vi "Remove Process.vi"(8 "error in (no error)":errorcluster, 10 "Process Name":string, 11 "Application In":refnum<class "Application.lvclass">) -> (0 "error out":errorcluster, 2 "App Process":refnum<class "Process.lvclass">, 3 "Application Out":refnum<class "Application.lvclass">)   [LabVIEW 2020, in "Application.lvclass"]
doc: "Get a specific process by name. A good pattern for using this VI is to wrap it with a string constant fed into the Process Name input and cast the received process to the expected process class. This pattern makes changing the class or the name easy as there is only one this single location where it is specified.\nThe VI can return processes from nested applications using the qualified name of the process."
uses:
  Application.lvclass
  C:/git/astemes-triarc-framework/source/Framework/Process/Process.lvclass
  Process/Process.lvclass
  C:/git/astemes-triarc-framework/source/Framework/Logging/Logging.lvclass
  Process/Process.lvclass/Process.ctl
  Application.lvclass/Application.ctl
  Process/Protected/Messaging/Request Message.vi
  <vilib>/AdvancedString/Delimited String to 1D String Array.vi
  Process/Protected/Messaging/Async Request Message.vi
  Process/Private/SubVIs/Handle Debug Data.vi
  Logging/Log Debug.vi
  <vilib>/AdvancedString/1D String Array to Delimited String.vi
  <vilib>/Utility/High Resolution Relative Seconds.vi
  Synchronous Request Callback/Synchronous Request Callback.lvclass
  C:/git/astemes-triarc-framework/source/Framework/Callback/Callback.lvclass
  <vilib>/Utility/error.llb/Error Cluster From Error Code.vi
  Synchronous Request Callback/Create.vi
  Process/Private/SubVIs/Wait for Response Message.vi
  Callback/Callback.lvclass
  Logging/Logging.lvclass
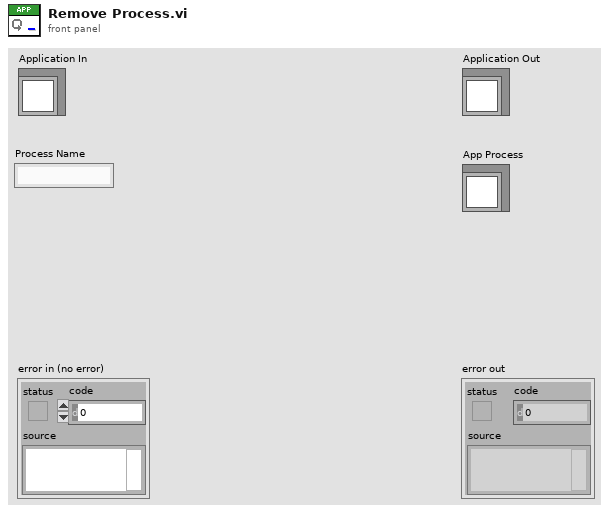
[diagram p1: front panel]
types:
  T1 = typedef "Process.lvclass/API Mode.ctl" = enum16{"Send Message", "Handle Message"}
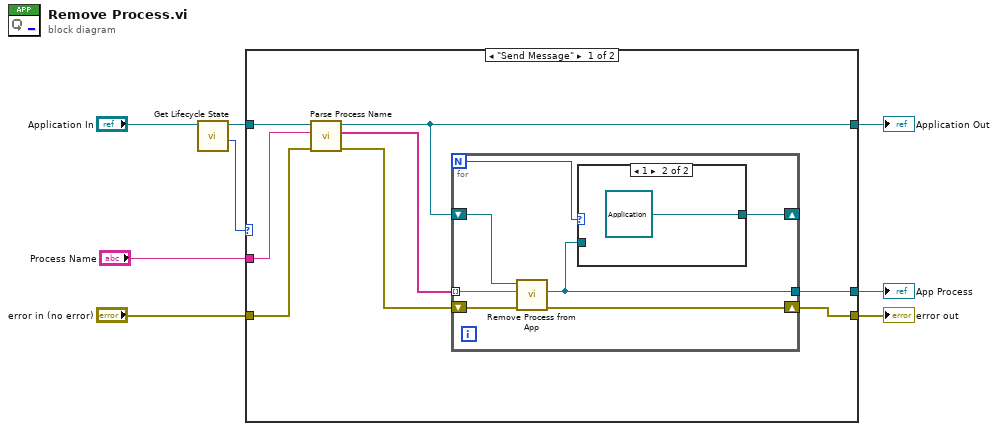
[diagram p0: block diagram]
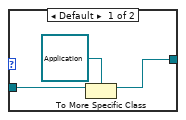
[diagram p2: hidden frame]
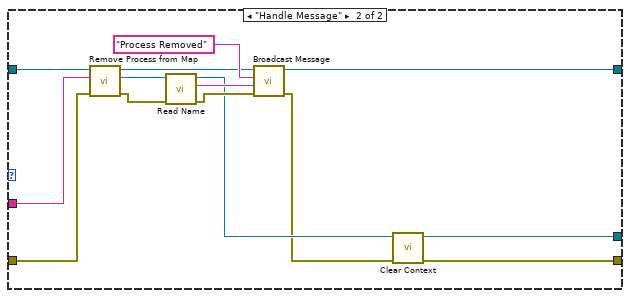
[diagram p3: hidden frame]
diagram:
  n1 = call "Get Lifecycle State.vi"("Process In"="Application In") -> ("API Mode"=w1:T1, "Process Out"=w2:refnum<class "Application.lvclass">)  [unwired: 7 in, 2 out]
  n2 = case shown="\"Send Message\"" w1 {
    tunnel: [w9 w31] -> w8
    tunnel: [w16 w28] -> w7
    tunnel: "Process Name" -> [w15 w41]
    tunnel: "error in (no error)" -> [w13 w32]
    tunnel: [w11 w35] -> w3
    tunnel: w2 -> [w10 w40]
    frame "Send Message" {
      n3 = call "Parse Process Name.vi"("error in (no error)"=w13, "Process Name"=w15, "Application In"=w10) -> ("error out"=w12:errorcluster, "Array"=w14:string[], "Application Out"=w11:refnum<class "Application.lvclass">)  [unwired: 6 in]
      n4 = for {
        N -> [w17]
        tunnel: [w19] -> w9
        tunnel: w14 -> [w21] mode=indexing
        shift-right: [w18] -> _
        shift-left: w11 -> [w22]
        shift-right: [w23] -> w16
        shift-left: w12 -> [w20]
        n5 = call "Remove Process from App.vi"("error in (no error)"=w20, "String"=w21, "Application In"=w22) -> ("error out"=w23:errorcluster, "Process"=w19:refnum<class "Process.lvclass">)  [unwired: 6 in, 1 out]
        n6 = case shown="1" w17 {
          tunnel: w19 -> [w26 _]
          tunnel: [w25 refnum<class "Application.lvclass"> refnum ("Application out")] -> w18
          frame Default {
            n7 = To More Specific Class(target class=refnum<class "Application.lvclass"> refnum ("Application out"), reference=w26) -> (specific class reference=w25:refnum<class "Application.lvclass">)  [unwired: 1 in, 1 out]
          }
          frame 1 {
          }
        }
      }
    }
    frame "Handle Message" {
      n8 = call "Remove Process from Map.vi"("error in (no error)"=w32, "Process Name"=w41, "Application In"=w40) -> ("error out"=w34:errorcluster, "Process"=w33:refnum<class "Process.lvclass">, "Application Out"=w36:refnum<class "Application.lvclass">)  [unwired: 6 in]
      n9 = call "Read Name.vi"("error in (no error)"=w34, "Process In"=w33) -> ("error out"=w38:errorcluster, "Qualified Name"=w37:string, "Process Out"=w30:refnum<class "Process.lvclass">)  [unwired: 6 in, 1 out]
      n10 = call-dynamic "Broadcast Message.vi"("error in (no error)"=w38, "Message Data"=w37, "Message"="Process Removed", "Process In"=w36) -> ("error out"=w29:errorcluster, "Process Out"=w35:refnum<class "Application.lvclass">)  [unwired: 6 in]
      n11 = call "Clear Context.vi"("error in (no error)"=w29, "Process In"=w30) -> ("error out"=w28:errorcluster, "Process Out"=w31:refnum<class "Process.lvclass">)  [unwired: 8 in]
    }
  }
  "error out" <- w7
  "Application Out" <- w3
  "App Process" <- w8
